vi "ReadBinaryWaveformFileOld.vi"(8 "error in (no error)":errorcluster, 9 "start of read offset (bytes:0)":i32, 11 "file path (dialog if empty)":path) -> (0 "error out":errorcluster, 1 "1D array":sgl[](array[numeric]) format="%.3f", 2 "2D array":sgl[][](array[numeric]) format="%.3f", 3 "new file path (Not A Path if cancelled)":path, 4 "EOF?":bool, 5 "mark after read (bytes)":i32, 6 "Time base":dbl format="%.2e", 7 "Delay, points":i32)   [LabVIEW 2015]
doc: "Reads a 2D or 1D array of data from a byte stream file of single-precision numbers (SGL). The VI opens the file beforehand and closes it afterwards. You can use this VI to read scaled data acquired from data acquisition VIs and written to a file with Write To SGL File.\n\nfile path is the path name of the file. If file path is empty (default value) or is Not A Path, the VI displays a File dialog box from which you can select a file. Error 43 occurs if the user cancels the dialog. \n\n¥ To read the entire file into 1D array, set 1D count <0 (default); you can leave 2D number of rows unwired.\n¥ To read N elements into 1D array, set 1D count =N and leave 2D number of rows wired or set to 0.\n¥ To read the entire file into 2D array, set 2D number of rows <0 and 2D number of columns =N >0. The VI calculates the number of rows as the integer part of file size/N.\n¥ To read M rows and N columns into 2D array, set 2D number of rows =M and 2D number of columns =N.\n\nstart of read offset is the position in the file, measured in bytes, at which the VI begins reading.\n\nnew file path is the path of the file from which the VI read data. You can use this output to determine the path of a file that you open using dialog. new file path returns Not A Path if the user selects Cancel from the dialog box.\n\n2D array contains the single precision numbers read from the file if 2D number of columns is >0 and 2D number of rows is <0 (meaning read the entire file) or >0 (read the the specified number of rows) ; otherwise, this output is empty.\n\n1D array contains the single precision numbers read from the file if 1D count is <0 (meaning read the entire file) or 2D number of rows =0 and 1D count is >0 (meaning read the specified number of samples); otherwise, this output is empty.\n\nmark after read is the location of the file mark after the read; it points to the byte in the file following the last byte read.\n\nEOF? is TRUE if you attempt to read past the end of file.\n\nRevisions:\n21 Oct 93: changes incorporated to read entire file (default to read entire file as 1D array); cosmetic changes.\n12 May 94: documentation changes."
panel:
  in  "prompt":string="Choose file to read."
  in  "instructions":string="* To read the entire file into 1D array, set 1D count <0 (default); you can leave 2D number of rows unwired.\n* To read N elements into 1D array, set 1D count =N and leave 2D number of rows wired or set to 0.\n* To read the entire file into 2D array, set 2D number of rows <0 and 2D number of columns =N >0.  The VI calculates the number of rows as the integer part of file size/N.\n* To read M rows and N columns into 2D array, set 2D number of rows =M and 2D number of columns =N."
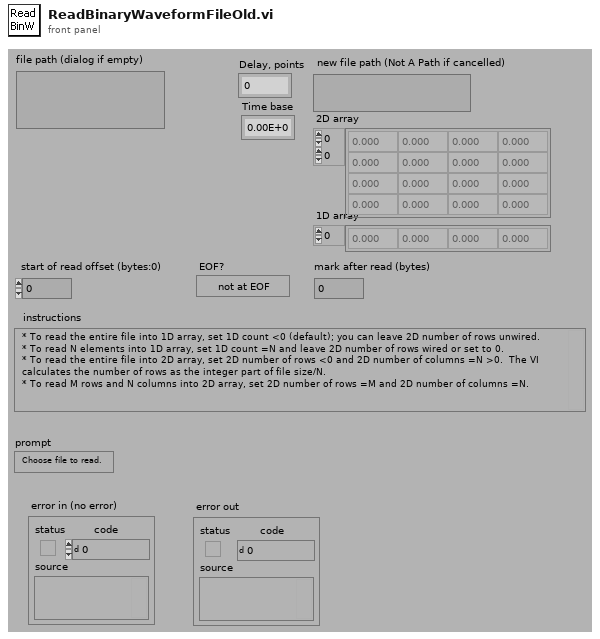
[diagram p1: front panel]
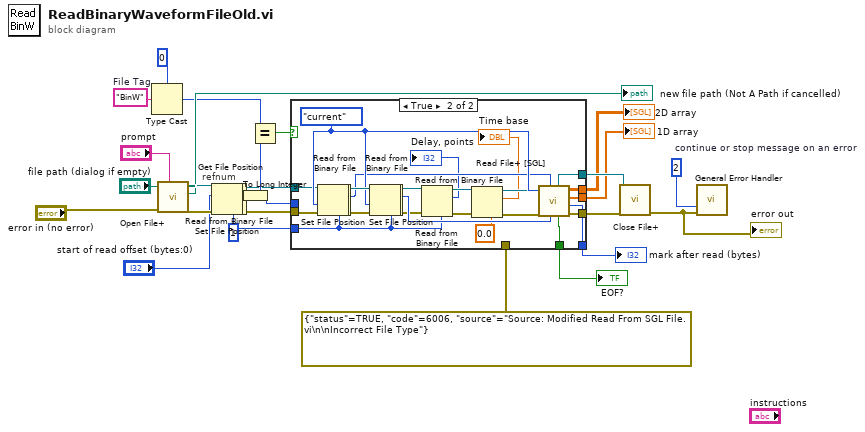
[diagram p0: block diagram]
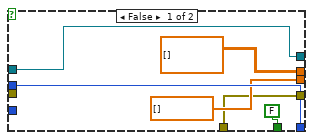
[diagram p2: hidden frame]
diagram:
  w8 = "BinW"  # File Tag
  w14 = 1 ("count")
  w29 = u16 2  # continue or stop message on an error
  # "error"
  # "refnum"
  n1 = Type Cast(type=0, x=w8) -> (*(type *) &x=w6:i32)
  n2 = call <vilib>:"Open File+.vi"("prompt"="prompt", "error in (not an error)"="error in (no error)", "file path (\" \")"="file path (dialog if empty)") -> ("error out"=w19:errorcluster, "file path"=→"new file path (Not A Path if cancelled)":path, "refnum"=w20:refnum<file>)  [unwired: 5 in, 1 out]
  n3 = Set File Position(offset (in bytes) (0)="start of read offset (bytes:0)", refnum=w20, error in=w19) -> (refnum out=w5:refnum<file>, error out=w4:errorcluster)  [unwired: 1 in]
  n4 = Read from Binary File(5:w14, 8:w4, 11:w5) -> (0:w2:errorcluster, 2:w18:i32, 3:w3:refnum<file>)  [unwired: 3 in, 1 out]
  n5 = Get File Position(4:w2, 7:w3) -> (0:w15:errorcluster, 2:w1:i64, 3:w16:refnum<file>)
  n6 = To Long Integer(number=w1) -> (32bit integer=w12:i32)
  n7 = Equal?(x=w6, y=w18) -> (x = y?=w17:bool)
  n8 = case shown="True" w17 {
    tunnel: [w31 w63] -> w28
    tunnel: [w36 w62] -> w27
    tunnel: [FALSE ("EOF?") w61] -> w26
    tunnel: [w32 w60] -> w25
    tunnel: [sgl[] [] ("1D data") w59] -> w24
    tunnel: [sgl[][] [] ("2D data") w58] -> w23
    tunnel: w16 -> [w32 w52]
    tunnel: w15 -> [_ w51]
    tunnel: w14 -> [_ w44]
    tunnel: w12 -> [w36 _]
    tunnel: errorcluster {"status"=TRUE, "code"=6006, "source"="Source: Modified Read From SGL File.vi\n\nIncorrect File Type"} ("error out") -> [w31 _]
    frame False {
    }
    frame True {
      w55 = enum16{"start", "end", "current"}."current" ("pos mode (0:2)")
      n9 = Set File Position(refnum=w52, from (0:start)=w55, error in=w51) -> (refnum out=w38:refnum<file>, error out=w37:errorcluster)  [unwired: 1 in]
      n10 = Read from Binary File(5:w44, 8:w37, 11:w38) -> (0:w57:errorcluster, 2:w53:i32, 3:w56:refnum<file>)  [unwired: 3 in, 1 out]
      n11 = Set File Position(refnum=w56, from (0:start)=w55, error in=w57) -> (refnum out=w40:refnum<file>, error out=w39:errorcluster)  [unwired: 1 in]
      n12 = Read from Binary File(5:w44, 8:w39, 11:w40) -> (0:w47:errorcluster, 2:w54:i32, 3:w50:refnum<file>)  [unwired: 3 in, 1 out]
      n13 = Read from Binary File(5:w44, 8:w47, 11:w50) -> (0:w46:errorcluster, 2:→"Delay, points":i32, 3:w49:refnum<file>)  [unwired: 3 in, 1 out]
      n14 = Read from Binary File(5:0.0, 8:w46, 11:w49) -> (0:w45:errorcluster, 2:→"Time base":dbl, 3:w48:refnum<file>)  [unwired: 3 in, 1 out]
      n15 = call <vilib>:"Read File+ [SGL].vi"("2D number of columns/1D count"=w54, "2D number of rows"=w53, "error in (no error)"=w45, "pos mode (rel. to current:2)"=w55, "refnum"=w48) -> ("error out"=w63:errorcluster, "mark after read (bytes)"=w62:i32, "1D data"=w59:sgl[], "2D data"=w58:sgl[][], "EOF?"=w61:bool, "dup refnum"=w60:refnum<file>)  [unwired: 1 in]
    }
  }
  "1D array" <- w24
  "mark after read (bytes)" <- w27
  "EOF?" <- w26
  "2D array" <- w23
  n16 = call <vilib>:"Close File+.vi"("error in (no error)"=w28, "refnum"=w25) -> ("error out"=w9:errorcluster)  [unwired: 3 in, 2 out]
  "error out" <- w9
  n17 = call <vilib>:"General Error Handler.vi"("type of dialog (OK msg:1)"=w29, "error in (no error)"=w9) -> ()  [unwired: 9 in, 5 out]
